vi "GaGeListDevices.vi"(8 "error in (no error)":errorcluster) -> (0 "error out":errorcluster, 3 "GaGe Boards":T1(array[cluster]))   [LabVIEW 2014]
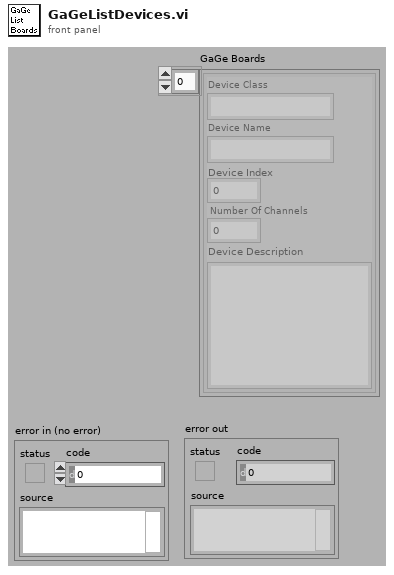
[diagram p1: front panel]
types:
  T1 = cluster{"Device Class":string, "Device Name":string, "Device Index":i32, "Number Of Channels":i32, "Device Description":string}[]
  T2 = cluster{"Handle":u32, "Sample size":u32, "Resolution":i32, "Offset":i32, "Channels":u32, "Boards":u32}
  T3 = cluster{string, "System Name":string, i32, i32, string}
  T4 = typedef "DAQ Settings.ctl" = cluster{"Timing for Groups":T5[], "Inputs":cluster{"Range":dbl, "Coupling":enum16{"Single", "Differen"}, "Impedance":dbl}[], "Trigger and sampling":cluster{"Trig. edge":enum16{"Rising", "Falling"}, "Trig. type":enum16{"Reference", "Immediate", "Start"}, "Trig. level":sgl, "Average samples":bool, "Oversample\nto match rates":bool}, "Integration":T6, "Temepature monitor":cluster{"Monitor temperature":bool, "Last T depth":i32, "Read rate, s":dbl, "Other GPIB instr's\n (\",\" separated)":refnum<visa-resource-name>[], "T-controller  VISA Name":refnum<visa-resource-name>}, "Device Array":cluster{cluster{"Device Name":string, "Number of channels":i32, "Device Index":i32, "Device type":enum16{"GaGe", "NI-DAQ", "NI-Scope", "CAMAC", "VXI-1433", "VXI-1437"}, "Total points":i64, "Current position":i64, "Chunk size":i64, "Active":bool, "Oversample by":i32, "Pre-trigger points":i64, "Fast mode":bool}[]}[], "NI-DAQ devices":cluster{"Clk source":string, "Trig. source":string, "Physical channels":string[], "sample mode":i32}[], "NI-Scope devices":cluster{"Channel names":string[], "trigger source":string, "Sample clock source":enum16{"Clock in", "None", "PXI star", "PFI 0", "PFI 1"}, "Sample Clock Timebase Divisor":i32}[], "CAMAC devices":cluster{"CAMAC\nGPIB address":string}, "HP 1433A devices":cluster{"Device Names":string}, "HP 1437A devices":cluster{"Device Names":string[]}, "File settings":T8, "Parameters":string, "DAQ State":cluster{"DAQ active":bool, "DAQ Armed":bool, "DAQ Triggered":bool}, "GaGe devices":cluster{"Mode":u16}[], "GaGe handles":cluster{"Handle":u32, "Sample size":u32, "Resolution":i32, "Offset":i32, "Channels":u32, "Boards":u32}[], "NI-Scope handles":refnum<k15>[], "NI-DAQ handles":refnum<k21>[], "T-controller object":refnum<class "Instrument.lvclass">, "End field value":dbl, "Local cell":string, "Trigger time":timestamp}
  T5 = typedef "Timing Element.ctl" = cluster{"Data rate":dbl, "Record length":dbl, "Pre-trigger length":dbl, "Ext. clock":bool}
  T6 = typedef "Integration.ctl" = cluster{"Offset duration, s":dbl, "Fix drift":bool, "Integrate channels":T7[]}
  T7 = typedef "Integrate channel.ctl" = cluster{"Channel":string, "Output name":string, "Factor":dbl}
  T8 = typedef "File settings.ctl" = cluster{"File Comments":string, "User/Prj":string, "Data folder":path, "File Index":enum16{"Local", "Cap Bank"}, "Time column":bool, "Save file":bool, "tdms file reference":refnum<k34>, "Settings file":path, "File Prefix":string, "Data file":path, "Channel names":string[], "Custom channel names":string[], "Column names":bool, "Disk space?":bool, "Generate ASCII":bool}
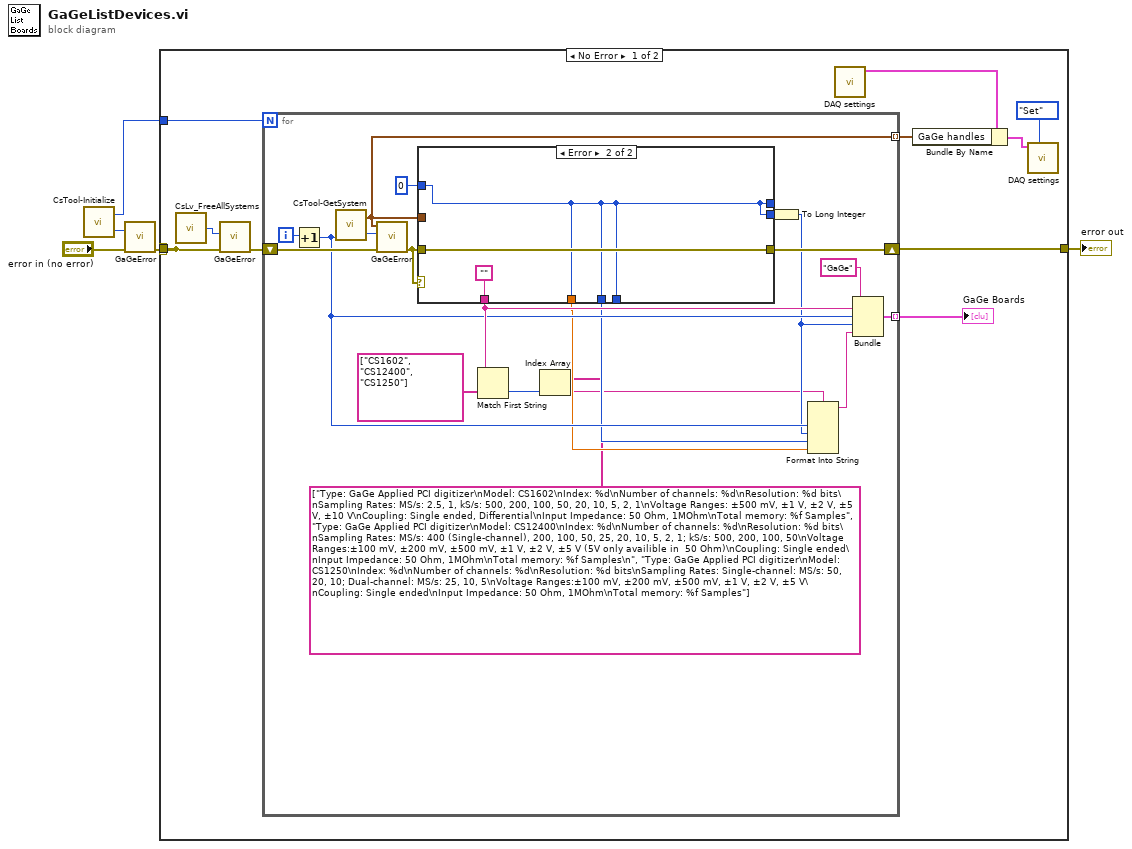
[diagram p0: block diagram]
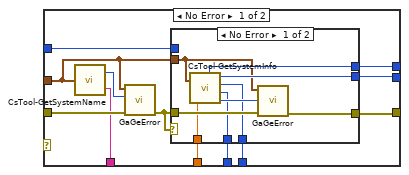
[diagram p2: hidden frame]
diagram:
  n1 = call "CsTool-Initialize.vi"() -> ("Error Code"=w5:i32, "Number Of Systems"=w3:i32)
  n2 = call "GaGeError.vi"("error in (no error)"="error in (no error)", "Error Code"=w5) -> ("error out"=w2:errorcluster)  [unwired: 4 in, 5 out]
  n3 = case shown="No Error" w2 {
    selector: w2 -> [w13 _]
    tunnel: w3 -> [w15 _]
    tunnel: w2 -> [_ w62]
    tunnel: [w9 w62] -> w1
    frame No Error {
      n4 = call "CsLv_FreeAllSystems.vi"() -> ("Error Code"=w11:i32)  [unwired: 1 out]
      n5 = call "GaGeError.vi"("error in (no error)"=w13, "Error Code"=w11) -> ("error out"=w12:errorcluster)  [unwired: 4 in, 5 out]
      n6 = for {
        N: w15 -> [_]
        shift-right: [w33] -> w9
        shift-left: w12 -> [w34]
        tunnel: [w30] -> w10 mode=indexing
        tunnel: [w23] -> w14 mode=indexing
        i -> [w29]
        n7 = Increment(x=w29) -> (x+1=w26:i32)
        n8 = call "CsTool-GetSystem.vi"("Index (0)"=w26) -> ("Error Code"=w35:i32, "Handle Cluster"=w30:T2)  [unwired: 3 in]
        n9 = call "GaGeError.vi"("error in (no error)"=w34, "Error Code"=w35, "Handle Cluster"=w30) -> ("error out"=w32:errorcluster)  [unwired: 3 in, 5 out]
        n10 = case shown="Error" w32 {
          tunnel: w32 -> [w47 w61]
          tunnel: [w46 w61] -> w33
          tunnel: w30 -> [w36 _]
          tunnel: [w43 ""] -> w27
          tunnel: [w42 w60] -> _
          tunnel: [w41 w60] -> w25
          tunnel: [w40 w60] -> _
          tunnel: [w39 w60] -> w21
          tunnel: [w38 w60] -> w20
          tunnel: u32 0 ("Board Type") -> [w37 w60]
          frame No Error {
            n11 = call "CsTool-GetSystemName.vi"("Handle Cluster"=w36) -> ("Error Code"=w44:i32, "System Name"=w43:string)
            n12 = call "GaGeError.vi"("error in (no error)"=w47, "Error Code"=w44, "Handle Cluster"=w36) -> ("error out"=w45:errorcluster)  [unwired: 3 in, 5 out]
            n13 = case shown="No Error" w45 {
              tunnel: w45 -> [w56 w58]
              tunnel: [w55 w58] -> w46
              tunnel: [w53 w57] -> w42
              tunnel: [w52 w57] -> w41
              tunnel: [w51 w57] -> w40
              tunnel: [w50 w57] -> w39
              tunnel: [w49 w57] -> w38
              tunnel: w37 -> [_ w57]
              tunnel: w36 -> [w48 _]
              frame No Error {
                n14 = call "CsTool-GetSystemInfo.vi"("Handle Cluster"=w48) -> ("Memory Size"=w49:dbl, "Board Type"=w53:u32, "Number Of Channels"=w52:u32, "Number Of Boards"=w51:u32, "Sample Bits"=w50:u32, "Error Code"=w54:i32)  [unwired: 1 out]
                n15 = call "GaGeError.vi"("error in (no error)"=w56, "Error Code"=w54, "Handle Cluster"=w48) -> ("error out"=w55:errorcluster)  [unwired: 3 in, 5 out]
              }
              frame Error {
              }
            }
          }
          frame Error {
          }
        }
        n16 = Match First String(2:string[] ["CS1602", "CS12400", "CS1250"], 3:w27) -> (0:w18:i32)  [unwired: 1 out]
        n17 = Index Array(array=string[] ["Type: GaGe Applied PCI digitizer\nModel: CS1602\nIndex: %d\nNumber of channels: %d\nResolution: %d bits\nSampling Rates: MS/s: 2.5, 1, kS/s: 500, 200, 100, 50, 20, 10, 5, 2, 1\nVoltage Ranges: ±500 mV, ±1 V, ±2 V, ±5 V, ±10 V\nCoupling: Single ended, Differential\nInput Impedance: 50 Ohm, 1MOhm\nTotal memory: %f Samples", "Type: GaGe Applied PCI digitizer\nModel: CS12400\nIndex: %d\nNumber of channels: %d\nResolution: %d bits\nSampling Rates: MS/s: 400 (Single-channel), 200, 100, 50, 25, 20, 10, 5, 2, 1; kS/s: 500, 200, 100, 50\nVoltage Ranges:±100 mV, ±200 mV, ±500 mV, ±1 V, ±2 V, ±5 V (5V only availible in  50 Ohm)\nCoupling: Single ended\nInput Impedance: 50 Ohm, 1MOhm\nTotal memory: %f Samples\n", "Type: GaGe Applied PCI digitizer\nModel: CS1250\nIndex: %d\nNumber of channels: %d\nResolution: %d bits\nSampling Rates: Single-channel: MS/s: 50, 20, 10; Dual-channel: MS/s: 25, 10, 5\nVoltage Ranges:±100 mV, ±200 mV, ±500 mV, ±1 V, ±2 V, ±5 V\nCoupling: Single ended\nInput Impedance: 50 Ohm, 1MOhm\nTotal memory: %f Samples"], index=w18) -> (element=w16:string)
        n18 = To Long Integer(number=w25) -> (32bit integer=w22:i32)
        n19 = Format Into String(format string=w16, w26, w22, w21, w20) -> (resulting string=w24:string)  [unwired: 2 in, 1 out]
        n20 = Bundle("GaGe", "System Name"=w27, w26, w22, w24) -> (w23:T3)  [unwired: 1 out]
      }
      "GaGe Boards" <- w14
      n21 = call "DAQ settings.vi"() -> ("DAQ Settings out"=w8:T4)  [unwired: 11 in]
      n22 = Bundle By Name(cluster=w8, "GaGe handles"=w10) -> (w7:T4)
      n23 = call "DAQ settings.vi"("Action"=enum16{"Get", "Set"}."Set", "DAQ Settings in"=w7) -> ()  [unwired: 9 in, 1 out]
    }
    frame Error {
    }
  }
  "error out" <- w1
